vi "Simulation Configuration Write.vi"(8 "error in (no error)":errorcluster, 10 "configuration":path=path "simulation configuration.ini", 11 "simulation configuration":T1={"maxTime"=5.0, "enableVisualization"=TRUE, "Environment Definition"=path "iRobot Navigation State Machine.vi", "Record Location"=path "Simulation Record.xml", "autograde?"=TRUE, "interactive?"=FALSE, "Feedback Mode"=enum."debug navigation", "Robot State Charts"=[path "C:/Users/blueuser/Desktop/Robo Sim Berkley/cpsgrader-release-0.4/Simulators/EECS149lab/src/LabVIEW/statechart/Simulation Statechart.vi"], "statechart"=path "C:/Users/blueuser/Desktop/Robo Sim Berkley/cpsgrader-release-0.4/Simulators/EECS149lab/src/LabVIEW/statechart/Simulation Statechart.vi"}) -> (0 "error out":errorcluster)   [LabVIEW 2015]
uses:
  CyberSim interface/Simulation Configuration.ctl
  autograder/feedbackMode.ctl
  <vilib>/Utility/config.llb/Write Key (Path).vi
  <vilib>/Utility/config.llb/Write Key (I32).vi
  <vilib>/Utility/config.llb/NI_LVConfig.lvlib
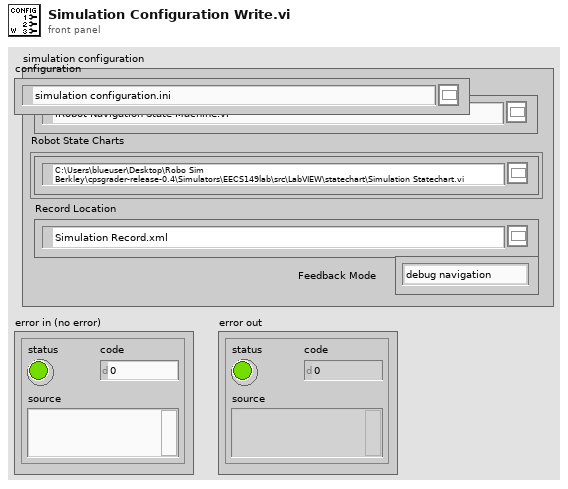
[diagram p1: front panel]
types:
  T1 = typedef "Simulation Configuration.ctl" = cluster{"maxTime":sgl, "enableVisualization":bool, "Environment Definition":path, "Record Location":path, "autograde?":bool, "interactive?":bool, "Feedback Mode":T2, "Robot State Charts":path[], "statechart":path}
  T2 = typedef "feedbackMode.ctl" = enum32{"debug navigation", "debug hill climb", "autograde navigation", "autograde hill climb"}
  T3 = typedef "NI_LVConfig.lvlib/Config Data RefNum.ctl" = refnum<k1>
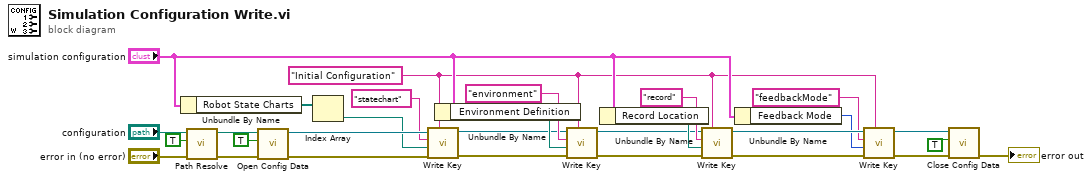
[diagram p0: block diagram]
diagram:
  w8 = "Initial Configuration" ("section")
  n1 = Unbundle By Name("simulation configuration") -> ("Robot State Charts"=w2:path[])
  n2 = call "Path Resolve.vi"("Error In"="error in (no error)", "create?"=TRUE, "absolute or relative path"="configuration") -> ("Error Out"=w20:errorcluster, "resolved path"=w21:path)  [unwired: 7 in]
  n3 = call <vilib>:"Open Config Data.vi"("error in (no error)"=w20, "create file if necessary (T)"=TRUE, "configuration file path"=w21) -> ("error out"=w28:errorcluster, "refnum"=w27:T3)  [unwired: 6 in, 1 out]
  n4 = Index Array(array=w2) -> (element=w1:path)  [unwired: 1 in]
  n5 = call-poly <vilib>:"Write Key.vi"("section"=w8, "error in (no error)"=w28, "value"=w1, "key"="statechart", "refnum"=w27) -> ("error out"=w16:errorcluster, "refnum out"=w17:T3)  [unwired: 4 in, 1 out]
  n6 = Unbundle By Name("simulation configuration") -> ("Environment Definition"=w25:path)
  n7 = call-poly <vilib>:"Write Key.vi"("section"=w8, "error in (no error)"=w16, "value"=w25, "key"="environment", "refnum"=w17) -> ("error out"=w4:errorcluster, "refnum out"=w5:T3)  [unwired: 4 in, 1 out]
  n8 = Unbundle By Name("simulation configuration") -> ("Record Location"=w14:path)
  n9 = call-poly <vilib>:"Write Key.vi"("section"=w8, "error in (no error)"=w4, "value"=w14, "key"="record", "refnum"=w5) -> ("error out"=w12:errorcluster, "refnum out"=w13:T3)  [unwired: 4 in, 1 out]
  n10 = Unbundle By Name("simulation configuration") -> ("Feedback Mode"=w10:T2)
  n11 = call-poly <vilib>:"Write Key.vi"("section"=w8, "error in (no error)"=w12, "value"=w10, "key"="feedbackMode", "refnum"=w13) -> ("error out"=w6:errorcluster, "refnum out"=w7:T3)  [unwired: 4 in, 1 out]
  n12 = call <vilib>:"Close Config Data.vi"("error in (no error)"=w6, "write file if changed (T)"=TRUE, "refnum"=w7) -> ("error out"=→"error out":errorcluster)  [unwired: 7 in, 1 out]
